vi "libssh2_session_method_pref.vi"(8 "error in (no error)":errorcluster, 9 "prefs":string, 10 "method_type":T1, 11 "session":T2) -> (0 "error out":errorcluster)   [LabVIEW 2013, in "libssh2.lvlib"]
doc: "Sets preferred methods to be negotiated. These preferences must be set prior to calling <B>libssh2_session_handshake</B> as they are used during the protocol initiation phase."
uses:
  libssh2.lvlib
  Session Refnum.ctl
  libssh2_method_type.ctl
  Not A Session.vi
  <vilib>/Utility/error.llb/Error Cluster From Error Code.vi
  Global Settings.vi
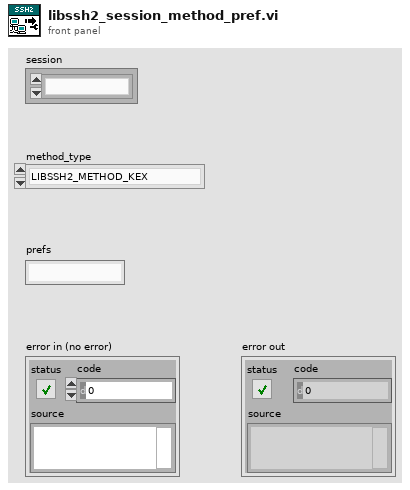
[diagram p1: front panel]
types:
  T1 = typedef "libssh2.lvlib/libssh2_method_type.ctl" = enum16{"LIBSSH2_METHOD_KEX", "LIBSSH2_METHOD_HOSTKEY", "LIBSSH2_METHOD_CRYPT_CS", "LIBSSH2_METHOD_CRYPT_SC", "LIBSSH2_METHOD_MAC_CS", "LIBSSH2_METHOD_MAC_SC", "LIBSSH2_METHOD_COMP_CS", "LIBSSH2_METHOD_COMP_SC", "LIBSSH2_METHOD_LANG_CS", "LIBSSH2_METHOD_LANG_SC", "LIBSSH2_METHOD_SIGN_ALGO"}
  T2 = typedef "libssh2.lvlib/Session Refnum.ctl" = refnum<k1>
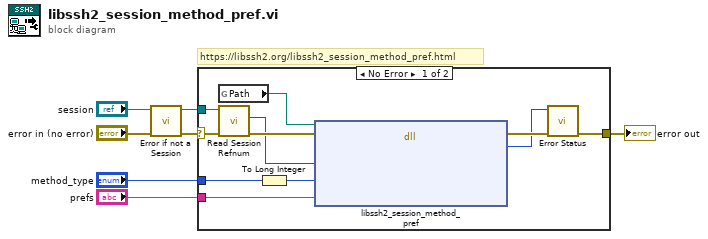
[diagram p0: block diagram]
diagram:
  # "https://libssh2.org/libssh2_session_method_pref.html"
  n1 = call "Error if not a Session.vi"("error in (no error)"="error in (no error)", "session"="session") -> ("error out"=w5:errorcluster, "session out"=w3:T2)  [unwired: 8 in]
  n2 = case shown="No Error" w5 {
    selector: w5 -> [w17 w19]
    tunnel: [w10 w19] -> w7
    tunnel: w3 -> [w16 _]
    tunnel: "method_type" -> [w12 _]
    tunnel: "prefs" -> [w8 _]
    frame No Error {
      n3 = global read "Global Settings.vi" "Path"() -> (w13:path)
      n4 = call "Read Session Refnum.vi"("error in (no error)"=w17, "session"=w16) -> ("error out"=w15:errorcluster, "LIBSSH2_SESSION*"=w14:u64)  [unwired: 8 in]
      n5 = To Long Integer(number=w12) -> (32bit integer=w11:i32)
      n6 = dll-call lib="?" fn="libssh2_session_method_pref"(path in=w13, error in=w15, "session"=w14, "method_type"=w11, "prefs"=w8) -> (error out=w18:errorcluster, "return value"=w9:i32)  [unwired: 4 in, 1 out]
      n7 = call "Error Status.vi"("error in (no error)"=w18, "return value"=w9) -> ("error out"=w10:errorcluster)  [unwired: 8 in, 1 out]
    }
    frame Error {
    }
  }
  "error out" <- w7
